vi "StringDateTimeToSQLDateTime.vi"(10 "String":string) -> (0 "time stamp":timestamp, 2 "date/time string":string)   [LabVIEW 2012]
uses:
  <vilib>/Utility/miscctls.llb/LVDateTimeRec.ctl
panel:
  in  "date time rec 2":T1
  out "output cluster":T1
  in  "date time rec":T1
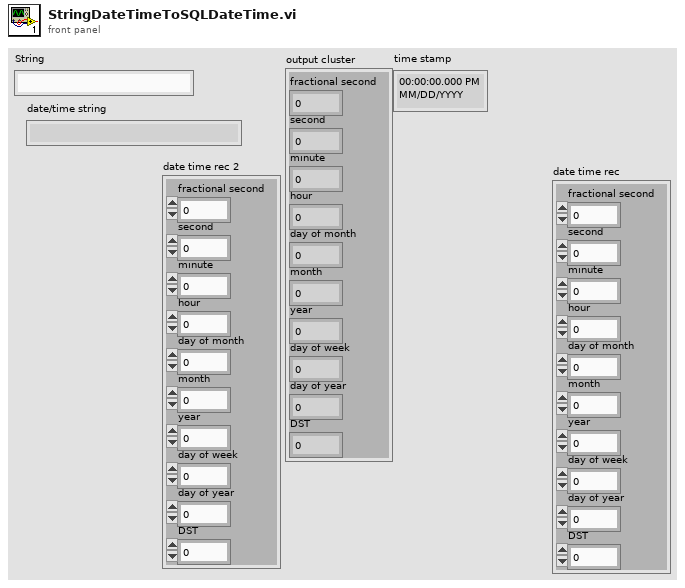
[diagram p1: front panel]
types:
  T1 = typedef "LVDateTimeRec.ctl" = cluster{"fractional second":dbl, "second":i32, "minute":i32, "hour":i32, "day of month":i32, "month":i32, "year":i32, "day of week":i32, "day of year":i32, "DST":i32}
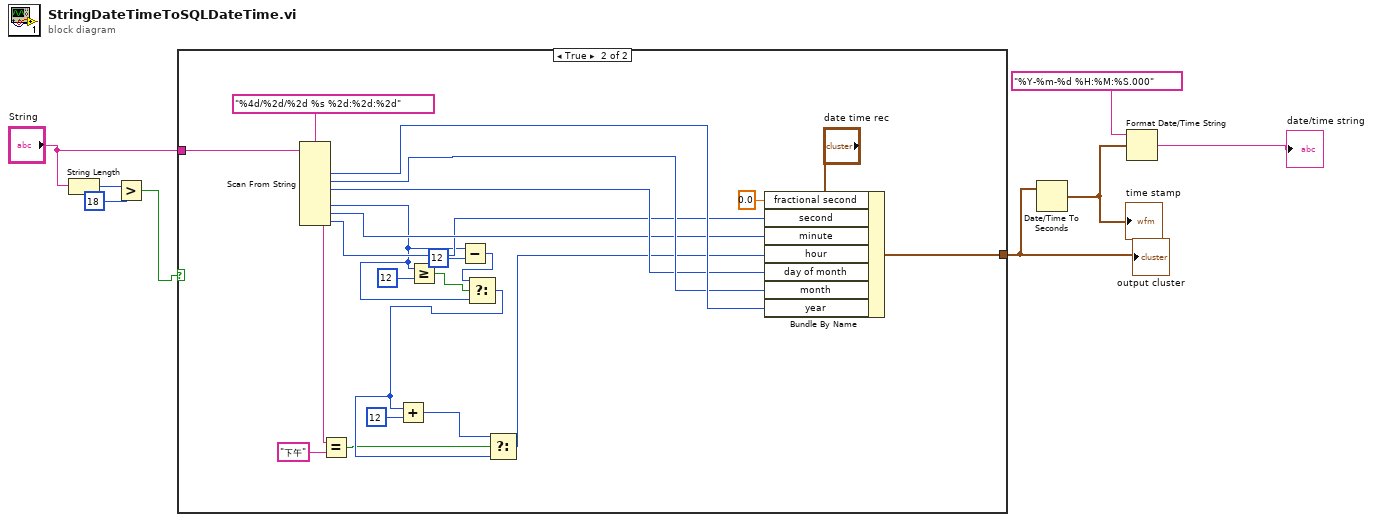
[diagram p0: block diagram]
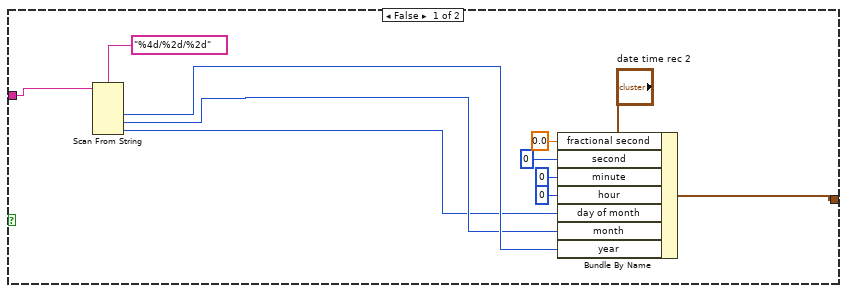
[diagram p2: hidden frame]
diagram:
  n1 = String Length(string="String") -> (length=w8:i32)
  n2 = Greater?(x=w8, y=18) -> (0:w6:bool)
  n3 = case shown="True" w6 {
    tunnel: "String" -> [w13 w28]
    tunnel: [w9 w27] -> w4
    frame False {
      n4 = Scan From String(format string="%4d/%2d/%2d", input string=w13) -> (output 1=w16:i32, output 2=w15:i32, output 3=w14:i32)  [unwired: 5 in, 3 out]
      n5 = Bundle By Name(cluster="date time rec 2", "fractional second"=0.0, "second"=0, "minute"=0, "hour"=0, "day of month"=w14, "month"=w15, "year"=w16) -> (w9:T1)
    }
    frame True {
      n6 = Scan From String(format string="%4d/%2d/%2d %s %2d:%2d:%2d", input string=w28) -> (output 1=w34:i32, output 2=w33:i32, output 3=w32:i32, output 4=w40:string, output 5=w24:i32, output 6=w30:i32, output 7=w29:i32)  [unwired: 9 in, 3 out]
      n7 = Equal?(x=w40, y="下午") -> (x = y?=w20:bool)
      n8 = Greater Or Equal?(x=w24, y=12) -> (x >= y?=w25:bool)
      n9 = Subtract(x=w24, y=12) -> (x-y=w22:i32)
      n10 = Select(t=w22, s=w25, f=w24) -> (s? t:f=w21:i32)
      n11 = Add(x=w21, y=12) -> (x+y=w37:i32)
      n12 = Select(t=w37, s=w20, f=w21) -> (s? t:f=w31:i32)
      n13 = Bundle By Name(cluster="date time rec", "fractional second"=0.0, "second"=w29, "minute"=w30, "hour"=w31, "day of month"=w32, "month"=w33, "year"=w34) -> (w27:T1)
    }
  }
  "output cluster" <- w4
  n14 = Date/Time To Seconds(2:w4) -> (0:w3:timestamp)  [unwired: 1 in]
  "time stamp" <- w3
  n15 = Format Date/Time String(time format string (%c)="%Y-%m-%d %H:%M:%S.000", seconds (now)=w3) -> (date/time string=→"date/time string":string)  [unwired: 1 in]
